vi "WriteSF.vi"(1 "Actuator ID\nBlue":u16=13, 4 "Actuator ID\nRed":u16=10, 7 "Motor value\nBlue":u8=50, 8 "connection IDs":T1={"Connected to\nsensors"=FALSE, "connection ID\nsensors"=refnum, "Connected to\nactuators"=TRUE, "connection ID\nactuators"=refnum}, 9 "Steering value\nBlue":u8, 11 "Motor value\nRed":u8=50, 13 "Steering value\nRed":u8=100) -> ()   [LabVIEW 2010]
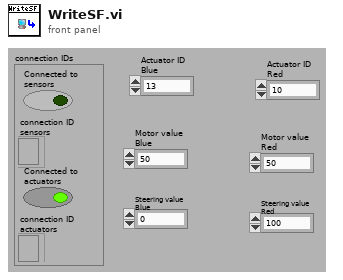
[diagram p1: front panel]
types:
  T1 = cluster{"Connected to\nsensors":bool, "connection ID\nsensors":refnum<k5>, "Connected to\nactuators":bool, "connection ID\nactuators":refnum<k5>}
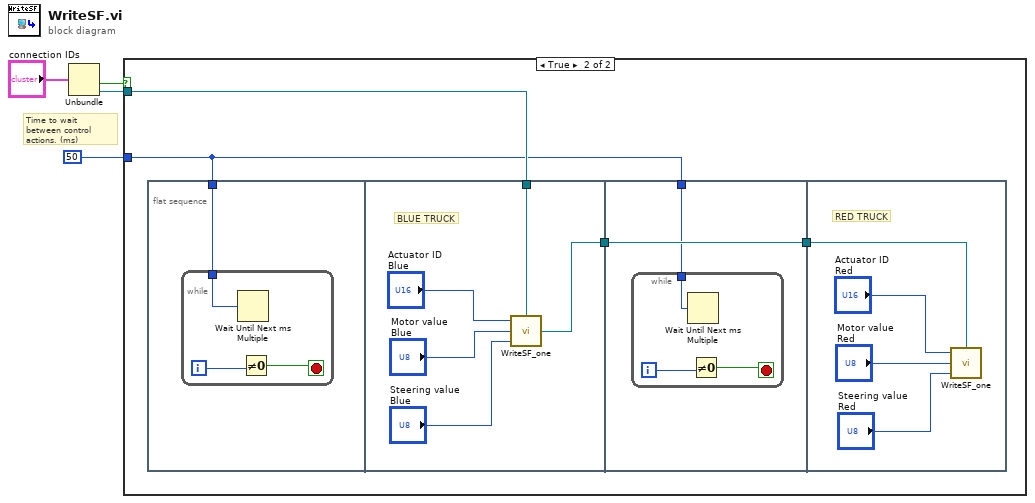
[diagram p0: block diagram]
diagram:
  # "Time to wait\nbetween control\nactions. (ms)"
  n1 = Unbundle("connection IDs") -> ("Connected to\nactuators"=w3:bool, "connection ID\nactuators"=w2:refnum<k5>)  [unwired: 2 out]
  n2 = case shown="True" w3 {
    tunnel: w2 -> [_ w8]
    tunnel: u32 50 ("millisecond multiple") -> [_ w5]
    frame False {
    }
    frame True {
      n3 = flat-sequence {
        tunnel: w5 -> [w9]
        tunnel: w8 -> [w14]
        tunnel: [w13] -> w7
        tunnel: w7 -> [w19]
        tunnel: [w19] -> w6
        tunnel: w5 -> [w18]
        tunnel: w6 -> [w26]
        frame #0 {
          n4 = while {
            tunnel: w9 -> [w10]
            i -> [w12]
            stop <- w11 stop-if-true
            n5 = Wait Until Next ms Multiple(millisecond multiple=w10) -> ()  [unwired: 1 out]
            n6 = Not Equal To 0?(x=w12) -> (x != 0?=w11:bool)
          }
        }
        frame #1 {
          # "BLUE TRUCK"
          n7 = call "WriteSF_one.vi"("connection ID in"=w14, "Steering value"="Steering value\nBlue", "Motor value"="Motor value\nBlue", "destination ID"="Actuator ID\nBlue") -> ("connection ID out"=w13:refnum<k5>)
        }
        frame #2 {
          n8 = while {
            tunnel: w18 -> [w20]
            i -> [w22]
            stop <- w21 stop-if-true
            n9 = Wait Until Next ms Multiple(millisecond multiple=w20) -> ()  [unwired: 1 out]
            n10 = Not Equal To 0?(x=w22) -> (x != 0?=w21:bool)
          }
        }
        frame #3 {
          # "RED TRUCK"
          n11 = call "WriteSF_one.vi"("connection ID in"=w26, "Steering value"="Steering value\nRed", "Motor value"="Motor value\nRed", "destination ID"="Actuator ID\nRed") -> ()  [unwired: 1 out]
        }
      }
    }
  }
